vi "createEngineeringList.vi"(8 "error in (no error)":errorcluster, 11 "ILCCommunications in":refnum<class "ILCCommunications.lvclass">) -> (0 "error out":errorcluster, 3 "ILCCommunications out":refnum<class "ILCCommunications.lvclass">)   [LabVIEW 2016, in "ILCCommunications.lvclass"]
uses:
  ILCCommunications.lvclass
  Common_RT_Modbus/ModbusBuffer/ModbusBuffer.lvclass
  Common_RT_Modbus/ModbusBuffer/ModbusBuffer.lvclass/ModbusBuffer.ctl
  ILCCommunications.lvclass/ILCCommunications.ctl
  Common_RT_ILC/ILC/ILC.lvclass/ILC.ctl
  Common_RT_FAILC/FAILC/FAILC.lvclass/FAILC.ctl
  Common_RT_HPILC/HPILC/HPILC.lvclass/HPILC.ctl
  Common_RT_Modbus/ModbusBuffer/writeSoftwareTrigger.vi
  Common_RT_Modbus/ModbusBuffer/writeHeader.vi
  Common_RT_FAILC/FAILC/startBroadcastSetForceFrame.vi
  Common_RT_ILC/ILC/getILCData.vi
  Common_RT_FAILC/FAILC/populateBroadcastSetForceFrame.vi
  Common_RT_FAILC/FAILC/completeBroadcastSetForceFrame.vi
  Common_RT_HPILC/HPILC/startBroadcastStepMotorFrame.vi
  Common_RT_HPILC/HPILC/populateBroadcastStepMotorFrame.vi
  Common_RT_HPILC/HPILC/completeBroadcastStepMotorFrame.vi
  Common_RT_Modbus/ModbusBuffer/writeTimestamp.vi
  reportFAForceAndStatus.vi
  reportHPForceAndStatus.vi
  reportHPServerStatus.vi
  Common_RT_Modbus/ModbusBuffer/writeTriggerIRQ.vi
  Common_RT_Modbus/ModbusBuffer/writeU8.vi
  Common_RT_FAILC/FAILC/determineSlewFlagValue.vi
  Common_RT_Modbus/ModbusBuffer/setIndex.vi
  Common_RT_Modbus/ModbusBuffer/writeI24.vi
  Common_RT_Modbus/ModbusBuffer/writeCRC.vi
  Common_RT_Modbus/ModbusBuffer/writeDelay.vi
  Common_RT_Modbus/ModbusBuffer/writeEndOfFrame.vi
  Common_RT_Modbus/ModbusBuffer/writeI8.vi
  Common_RT_FAILC/FAILC/addForceAndStatusFrame.vi
  Common_RT_HPILC/HPILC/createForceAndStatusFrame.vi
  reportServerStatus.vi
  Common_RT_Modbus/ModbusBuffer/writeByteInstruction.vi
  Common_RT_Modbus/ModbusBuffer/calculateCRC.vi
  Common_RT_Modbus/ModbusBuffer/writeWaitForRx.vi
  Common_RT_ILC/ILC/addReportServerStatusFrame.vi
  Common_RT_FAILC/FAILC/FAILC.lvclass
  D:/Code/ts_M1M3Support/Common_RT_ILC/ILC/ILC.lvclass
  Common_RT_HPILC/HPILC/HPILC.lvclass
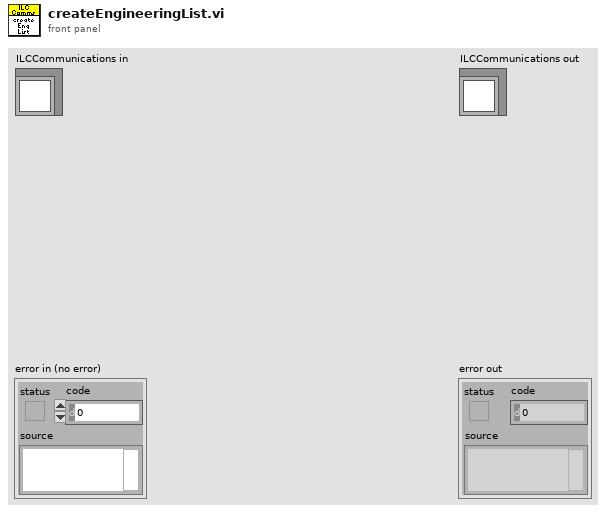
[diagram p1: front panel]
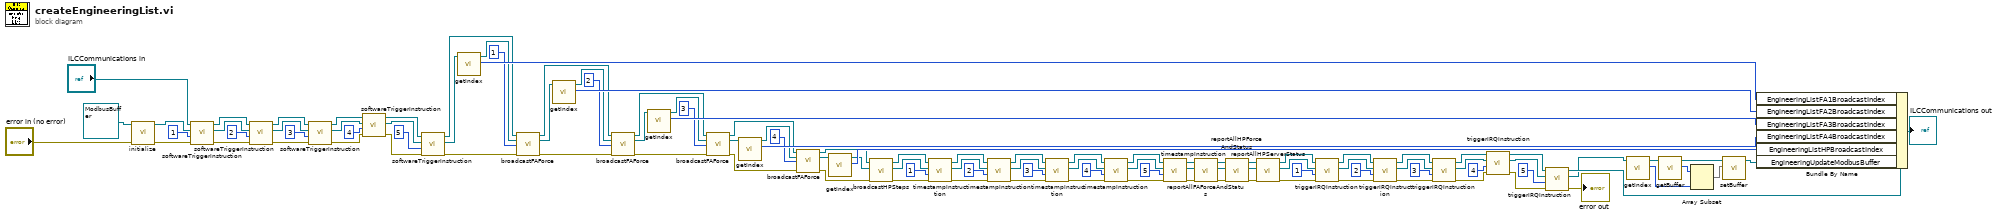
[diagram p0: block diagram]
diagram:
  n1 = call "initialize.vi"("error in (no error)"="error in (no error)", "ModbusBuffer in"=refnum<class "ModbusBuffer.lvclass"> refnum ("RTModbus.lvlib:ModbusBuffer.lvclass")) -> ("error out"=w81:errorcluster, "ModbusBuffer out"=w86:refnum<class "ModbusBuffer.lvclass">)  [unwired: 8 in]
  n2 = call "softwareTriggerInstruction.vi"("error in (no error)"=w81, "Subnet"=u8 1, "ModbusBuffer in"=w86, "ILCCommunications in"="ILCCommunications in") -> ("error out"=w80:errorcluster, "ModbusBuffer out"=w85:refnum<class "ModbusBuffer.lvclass">, "ILCCommunications out"=w90:refnum<class "ILCCommunications.lvclass">)  [unwired: 5 in]
  n3 = call "softwareTriggerInstruction.vi"("error in (no error)"=w80, "Subnet"=u8 2, "ModbusBuffer in"=w85, "ILCCommunications in"=w90) -> ("error out"=w79:errorcluster, "ModbusBuffer out"=w84:refnum<class "ModbusBuffer.lvclass">, "ILCCommunications out"=w89:refnum<class "ILCCommunications.lvclass">)  [unwired: 5 in]
  n4 = call "softwareTriggerInstruction.vi"("error in (no error)"=w79, "Subnet"=u8 3, "ModbusBuffer in"=w84, "ILCCommunications in"=w89) -> ("error out"=w78:errorcluster, "ModbusBuffer out"=w83:refnum<class "ModbusBuffer.lvclass">, "ILCCommunications out"=w88:refnum<class "ILCCommunications.lvclass">)  [unwired: 5 in]
  n5 = call "softwareTriggerInstruction.vi"("error in (no error)"=w78, "Subnet"=u8 4, "ModbusBuffer in"=w83, "ILCCommunications in"=w88) -> ("error out"=w77:errorcluster, "ModbusBuffer out"=w82:refnum<class "ModbusBuffer.lvclass">, "ILCCommunications out"=w87:refnum<class "ILCCommunications.lvclass">)  [unwired: 5 in]
  n6 = call "softwareTriggerInstruction.vi"("error in (no error)"=w77, "Subnet"=u8 5, "ModbusBuffer in"=w82, "ILCCommunications in"=w87) -> ("error out"=w20:errorcluster, "ModbusBuffer out"=w92:refnum<class "ModbusBuffer.lvclass">, "ILCCommunications out"=w26:refnum<class "ILCCommunications.lvclass">)  [unwired: 5 in]
  n7 = call "getIndex.vi"("ModbusBuffer in"=w92) -> ("Index"=w50:i32, "ModbusBuffer out"=w14:refnum<class "ModbusBuffer.lvclass">)  [unwired: 9 in]
  n8 = call "broadcastFAForce.vi"("ILCCommunications in"=w26, "ModbusBuffer in"=w14, "Subnet"=u8 1, "error in (no error)"=w20) -> ("ILCCommunications out"=w25:refnum<class "ILCCommunications.lvclass">, "ModbusBuffer out"=w13:refnum<class "ModbusBuffer.lvclass">, "error out"=w19:errorcluster)  [unwired: 9 in]
  n9 = call "getIndex.vi"("ModbusBuffer in"=w13) -> ("Index"=w49:i32, "ModbusBuffer out"=w12:refnum<class "ModbusBuffer.lvclass">)  [unwired: 9 in]
  n10 = call "broadcastFAForce.vi"("ILCCommunications in"=w25, "ModbusBuffer in"=w12, "Subnet"=u8 2, "error in (no error)"=w19) -> ("ILCCommunications out"=w24:refnum<class "ILCCommunications.lvclass">, "ModbusBuffer out"=w11:refnum<class "ModbusBuffer.lvclass">, "error out"=w18:errorcluster)  [unwired: 9 in]
  n11 = call "getIndex.vi"("ModbusBuffer in"=w11) -> ("Index"=w48:i32, "ModbusBuffer out"=w10:refnum<class "ModbusBuffer.lvclass">)  [unwired: 9 in]
  n12 = call "broadcastFAForce.vi"("ILCCommunications in"=w24, "ModbusBuffer in"=w10, "Subnet"=u8 3, "error in (no error)"=w18) -> ("ILCCommunications out"=w23:refnum<class "ILCCommunications.lvclass">, "ModbusBuffer out"=w9:refnum<class "ModbusBuffer.lvclass">, "error out"=w17:errorcluster)  [unwired: 9 in]
  n13 = call "getIndex.vi"("ModbusBuffer in"=w9) -> ("Index"=w47:i32, "ModbusBuffer out"=w8:refnum<class "ModbusBuffer.lvclass">)  [unwired: 9 in]
  n14 = call "broadcastFAForce.vi"("ILCCommunications in"=w23, "ModbusBuffer in"=w8, "Subnet"=u8 4, "error in (no error)"=w17) -> ("ILCCommunications out"=w22:refnum<class "ILCCommunications.lvclass">, "ModbusBuffer out"=w7:refnum<class "ModbusBuffer.lvclass">, "error out"=w16:errorcluster)  [unwired: 9 in]
  n15 = call "getIndex.vi"("ModbusBuffer in"=w7) -> ("Index"=w46:i32, "ModbusBuffer out"=w6:refnum<class "ModbusBuffer.lvclass">)  [unwired: 9 in]
  n16 = call "broadcastHPSteps.vi"("error in (no error)"=w16, "ModbusBuffer in"=w6, "ILCCommunications in"=w22) -> ("error out"=w15:errorcluster, "ModbusBuffer out"=w5:refnum<class "ModbusBuffer.lvclass">, "ILCCommunications out"=w21:refnum<class "ILCCommunications.lvclass">)  [unwired: 6 in]
  n17 = call "timestampInstruction.vi"("error in (no error)"=w15, "Subnet"=u8 1, "ModbusBuffer in"=w5, "ILCCommunications in"=w21) -> ("error out"=w64:errorcluster, "ModbusBuffer out"=w68:refnum<class "ModbusBuffer.lvclass">, "ILCCommunications out"=w72:refnum<class "ILCCommunications.lvclass">)  [unwired: 5 in]
  n18 = call "timestampInstruction.vi"("error in (no error)"=w64, "Subnet"=u8 2, "ModbusBuffer in"=w68, "ILCCommunications in"=w72) -> ("error out"=w63:errorcluster, "ModbusBuffer out"=w67:refnum<class "ModbusBuffer.lvclass">, "ILCCommunications out"=w71:refnum<class "ILCCommunications.lvclass">)  [unwired: 5 in]
  n19 = call "timestampInstruction.vi"("error in (no error)"=w63, "Subnet"=u8 3, "ModbusBuffer in"=w67, "ILCCommunications in"=w71) -> ("error out"=w62:errorcluster, "ModbusBuffer out"=w66:refnum<class "ModbusBuffer.lvclass">, "ILCCommunications out"=w70:refnum<class "ILCCommunications.lvclass">)  [unwired: 5 in]
  n20 = call "timestampInstruction.vi"("error in (no error)"=w62, "Subnet"=u8 4, "ModbusBuffer in"=w66, "ILCCommunications in"=w70) -> ("error out"=w61:errorcluster, "ModbusBuffer out"=w65:refnum<class "ModbusBuffer.lvclass">, "ILCCommunications out"=w69:refnum<class "ILCCommunications.lvclass">)  [unwired: 5 in]
  n21 = call "timestampInstruction.vi"("error in (no error)"=w61, "Subnet"=u8 5, "ModbusBuffer in"=w65, "ILCCommunications in"=w69) -> ("error out"=w51:errorcluster, "ModbusBuffer out"=w54:refnum<class "ModbusBuffer.lvclass">, "ILCCommunications out"=w56:refnum<class "ILCCommunications.lvclass">)  [unwired: 5 in]
  n22 = call "reportAllFAForceAndStatus.vi"("error in (no error)"=w51, "ModbusBuffer in"=w54, "ILCCommunications in"=w56) -> ("error out"=w52:errorcluster, "ModbusBuffer out"=w53:refnum<class "ModbusBuffer.lvclass">, "ILCCommunications out"=w55:refnum<class "ILCCommunications.lvclass">)  [unwired: 6 in]
  n23 = call "reportAllHPForceAndStatus.vi"("error in (no error)"=w52, "ModbusBuffer in"=w53, "ILCCommunications in"=w55) -> ("error out"=w103:errorcluster, "ModbusBuffer out"=w109:refnum<class "ModbusBuffer.lvclass">, "ILCCommunications out"=w110:refnum<class "ILCCommunications.lvclass">)  [unwired: 6 in]
  n24 = call "reportAllHPServerStatus.vi"("error in (no error)"=w103, "ModbusBuffer in"=w109, "ILCCommunications in"=w110) -> ("error out"=w35:errorcluster, "ModbusBuffer out"=w40:refnum<class "ModbusBuffer.lvclass">, "ILCCommunications out"=w45:refnum<class "ILCCommunications.lvclass">)  [unwired: 6 in]
  n25 = call "triggerIRQInstruction.vi"("error in (no error)"=w35, "Subnet"=u8 1, "ModbusBuffer in"=w40, "ILCCommunications in"=w45) -> ("error out"=w34:errorcluster, "ModbusBuffer out"=w39:refnum<class "ModbusBuffer.lvclass">, "ILCCommunications out"=w44:refnum<class "ILCCommunications.lvclass">)  [unwired: 5 in]
  n26 = call "triggerIRQInstruction.vi"("error in (no error)"=w34, "Subnet"=u8 2, "ModbusBuffer in"=w39, "ILCCommunications in"=w44) -> ("error out"=w33:errorcluster, "ModbusBuffer out"=w38:refnum<class "ModbusBuffer.lvclass">, "ILCCommunications out"=w43:refnum<class "ILCCommunications.lvclass">)  [unwired: 5 in]
  n27 = call "triggerIRQInstruction.vi"("error in (no error)"=w33, "Subnet"=u8 3, "ModbusBuffer in"=w38, "ILCCommunications in"=w43) -> ("error out"=w32:errorcluster, "ModbusBuffer out"=w37:refnum<class "ModbusBuffer.lvclass">, "ILCCommunications out"=w42:refnum<class "ILCCommunications.lvclass">)  [unwired: 5 in]
  n28 = call "triggerIRQInstruction.vi"("error in (no error)"=w32, "Subnet"=u8 4, "ModbusBuffer in"=w37, "ILCCommunications in"=w42) -> ("error out"=w31:errorcluster, "ModbusBuffer out"=w36:refnum<class "ModbusBuffer.lvclass">, "ILCCommunications out"=w41:refnum<class "ILCCommunications.lvclass">)  [unwired: 5 in]
  n29 = call "triggerIRQInstruction.vi"("error in (no error)"=w31, "Subnet"=u8 5, "ModbusBuffer in"=w36, "ILCCommunications in"=w41) -> ("error out"=→"error out":errorcluster, "ModbusBuffer out"=w97:refnum<class "ModbusBuffer.lvclass">, "ILCCommunications out"=w99:refnum<class "ILCCommunications.lvclass">)  [unwired: 5 in]
  n30 = call "getIndex.vi"("ModbusBuffer in"=w97) -> ("Index"=w107:i32, "ModbusBuffer out"=w106:refnum<class "ModbusBuffer.lvclass">)  [unwired: 9 in]
  n31 = call "getBuffer.vi"("ModbusBuffer in"=w106) -> ("Buffer"=w108:u16[], "ModbusBuffer out"=w104:refnum<class "ModbusBuffer.lvclass">)  [unwired: 9 in]
  n32 = Array Subset(array=w108, length=w107) -> (w105:u16[])  [unwired: 1 in]
  n33 = call "setBuffer.vi"("Buffer"=w105, "ModbusBuffer in"=w104) -> ("ModbusBuffer out"=w101:refnum<class "ModbusBuffer.lvclass">)  [unwired: 9 in]
  n34 = Bundle By Name(cluster=w99, "EngineeringListFA1BroadcastIndex"=w50, "EngineeringListFA2BroadcastIndex"=w49, "EngineeringListFA3BroadcastIndex"=w48, "EngineeringListFA4BroadcastIndex"=w47, "EngineeringListHPBroadcastIndex"=w46, "EngineeringUpdateModbusBuffer"=w101) -> (→"ILCCommunications out":refnum<class "ILCCommunications.lvclass">)
